vi "binary_string.vi"() -> ()   [LabVIEW 2021]
panel:
  out "data":i8[](array[numeric])
  out "path":path
  out "error out":errorcluster
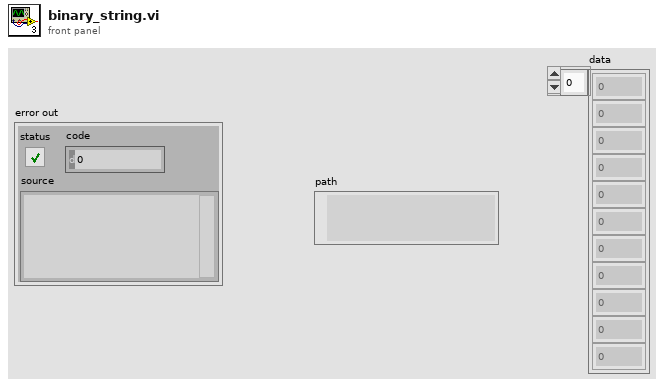
[diagram p1: front panel]
types:
  T1 = enum16{"open", "replace", "create", "open or create", "replace or create", "replace or create with confirmation"}
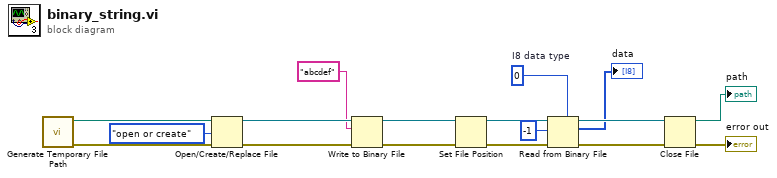
[diagram p0: block diagram]
diagram:
  w2 = i8 0  # I8 data type
  n1 = call <vilib>:"Generate Temporary File Path.vi"() -> ("error out"=w9:errorcluster, "Unique Temporary File Path"=w10:path)  [unwired: 10 in]
  n2 = Open/Create/Replace File(file path (use dialog)=w10, error in=w9, operation (0:open)=T1."open or create") -> (refnum out=w7:refnum<file>, error out=w8:errorcluster)  [unwired: 3 in, 1 out]
  n3 = Write to Binary File(file (use dialog)=w7, data="abcdef", error in=w8) -> (refnum out=w15:refnum<file>, error out=w13:errorcluster)  [unwired: 3 in, 1 out]
  n4 = Set File Position(refnum=w15, error in=w13) -> (refnum out=w14:refnum<file>, error out=w12:errorcluster)  [unwired: 2 in]
  n5 = Read from Binary File(5:w2, 8:w12, 10:-1 ("count (1)"), 11:w14) -> (0:w16:errorcluster, 2:→"data":i8[], 3:w17:refnum<file>)  [unwired: 2 in, 1 out]
  n6 = Close File(refnum=w17, error in=w16) -> (path=→"path":path, error out=→"error out":errorcluster)
